vi "Teardown.vi"(6 "Error":errorcluster, 7 "Actor":refnum<class "Actor Layer.lvclass">, 9 "UnhandledMsgs":refnum<class "Msg.lvclass">[](array[class]), 10 "UnhandledMsgAttribs":T1[](array[typedef]) {"Listen Absolute Time" format="%<%x %.3X>T"; "Tell Absolute Time" format="%<%x %.3X>T"}) -> ()   [LabVIEW 2020, in "_Template.lvlib" / "{{Actor}}.lvlib" / "Actor Layer.lvclass"]
uses:
  Actor Layer.lvclass
  Actor Layer.lvclass/Actor Layer.ctl
  jettl/jettl/Actor Layer/Actor Layer.lvclass
  jettl/jettl/Msg/Msg.lvclass
  jettl/jettl/Origin.ctl
  jettl/jettl/jettl.lvlib
  jettl/jettl/Lifecycle.ctl
  jettl/jettl/Msg Execute Type.ctl
  jettl/jettl/Msg Attribs.ctl
panel:
  # "This front panel should not be manipulated."
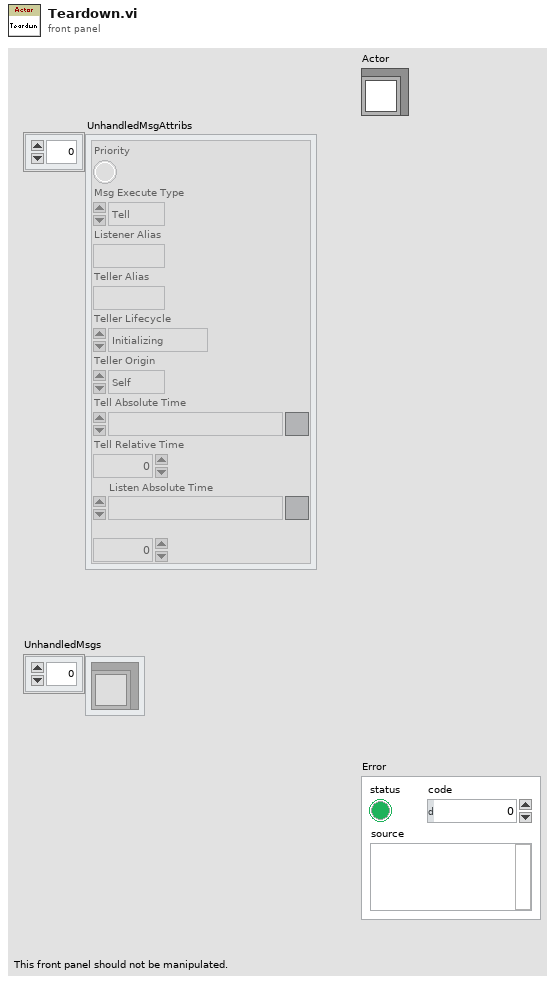
[diagram p1: front panel]
types:
  T1 = typedef "jettl.lvlib/Msg Attribs.ctl" = cluster{"Priority":bool, "Msg Execute Type":T2, "Listener Alias":string, "Teller Alias":string, "Teller Lifecycle":T3, "Teller Origin":T4, "Tell Absolute Time":timestamp, "Tell Relative Time":dbl, "Listen Absolute Time":timestamp, "Listen Relative Time":dbl}
  T2 = typedef "jettl.lvlib/Msg Execute Type.ctl" = enum16{"Tell", "Call"}
  T3 = typedef "jettl.lvlib/Lifecycle.ctl" = enum16{"Initializing", "Setting Up", "Starting", "Running", "Stopping", "Tearing Down", "Terminated"}
  T4 = typedef "jettl.lvlib/Origin.ctl" = enum16{"Self", "Parent", "Child"}
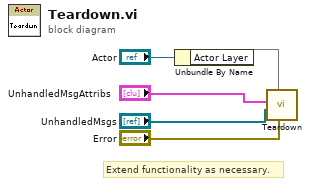
[diagram p0: block diagram]
diagram:
  # "Extend functionality as necessary."
  n1 = Unbundle By Name("Actor") -> ("Actor Layer"=w3)
  n2 = call-dynamic "Teardown.vi"("Error"="Error", "Actor"=w3, "UnhandledMsgs"="UnhandledMsgs", "UnhandledMsgAttribs"="UnhandledMsgAttribs") -> ()  [unwired: 6 in, 2 out]
